vi "LIF V3.0.vi"() -> ()   [LabVIEW 2022 SP3]
uses:
  <vilib>/Utility/error.llb/DialogType.ctl
  <vilib>/DAQmx/read.llb/DAQmx Read (Analog 1D DBL 1Chan NSamp).vi
  <vilib>/DAQmx/create/channels.llb/DAQmx Create Channel (AI-Voltage-Basic).vi
  <vilib>/DAQmx/miscellaneous.llb/DAQmx Fill In Error Info.vi
  Instance           6 23Saved   Maxium LIF V2.0 .vi
  Instance           7 23Saved   Maxium LIF V2.0 .vi
  Instance           3 23Saved   Maxium LIF V2.0 .vi
panel:
  in  "Number of Samples to Average":i32=500
  out "Time Remaining":dbl format="%<%H:%M:%S>t"
  out "Scanning?":bool
  out "file ref":refnum<file>
  out "Sample X data":dbl[](array[numeric])
  out "sample Y data":dbl[](array[numeric])
  in  "STOP":bool
  out "Current Position (cm-1)":dbl format="%.3f"
  in  "Experimental Conditions":string
  in  "Time to wait (s)":dbl=6.0 min=0.0 max=60.0
  in  "Step Size (cm-1)":dbl=0.003 min=0.001 max=10.0 step=0.001 format="%.3f"
  in  "End Position (cm-1)":dbl=650.3 min=0.0 max=2000.0 step=0.001 format="%.3f"
  in  "Start Position (cm-1)":dbl min=0.0 max=0.0 step=0.001 format="%.3f"
  out "LIF Spectrum":cluster{"Y":dbl[], "Y":dbl[]}[](graph)
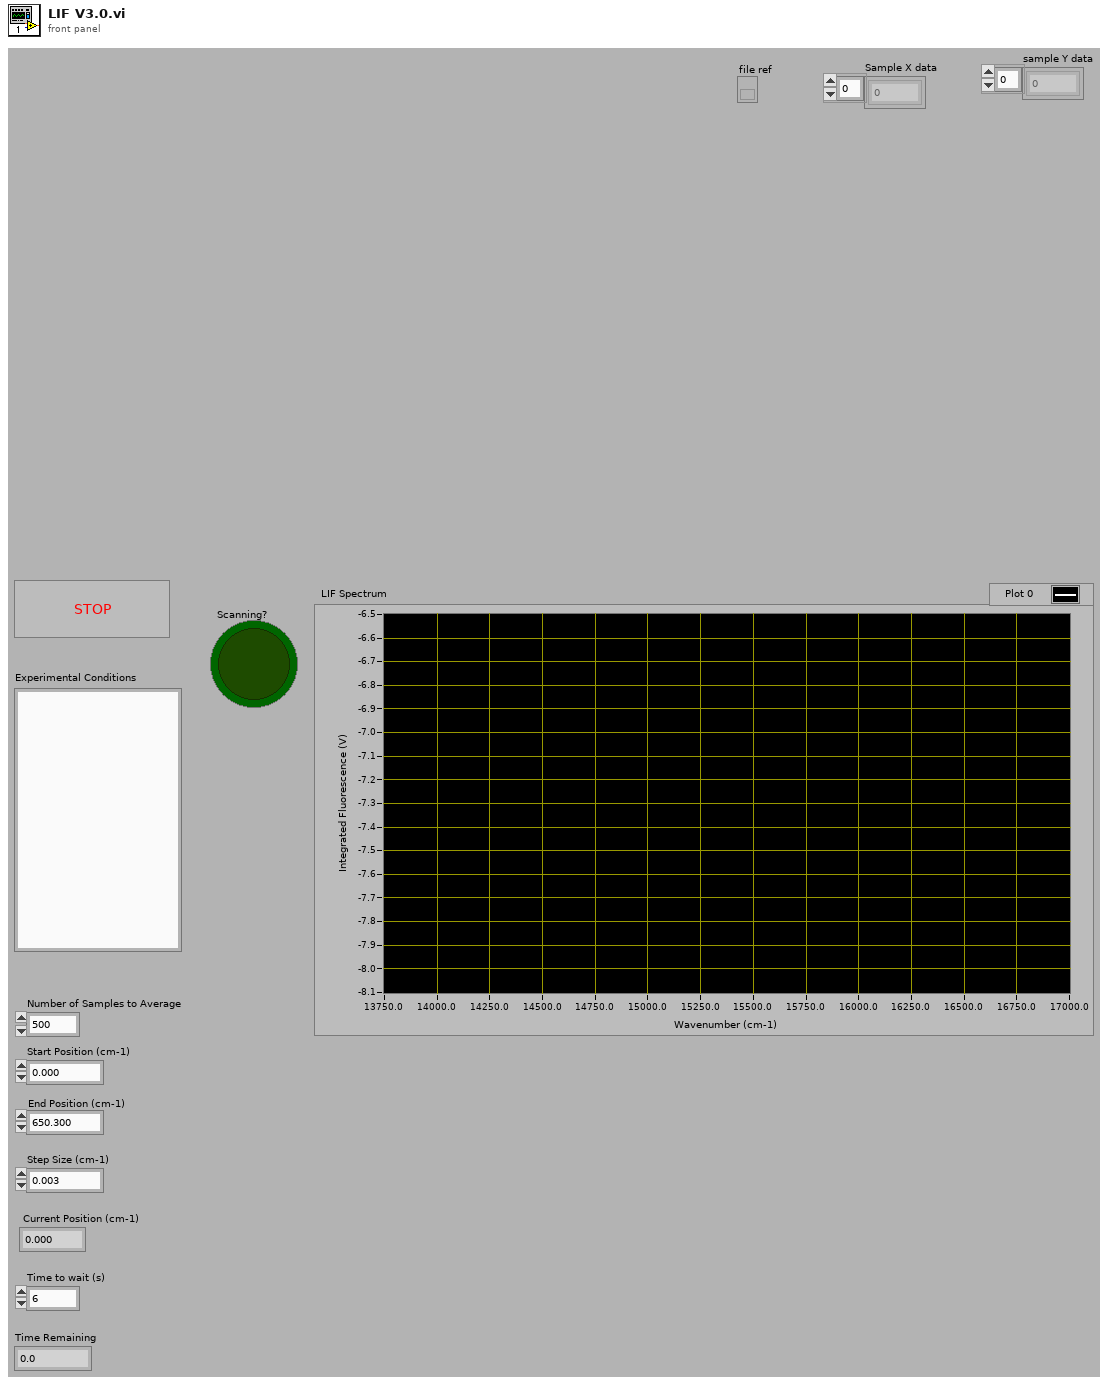
[diagram p1: front panel]
types:
  T1 = typedef "DialogType.ctl" = u16
  T2 = enum16{"open", "open or create", "create or replace", "create", "open (read only)"}
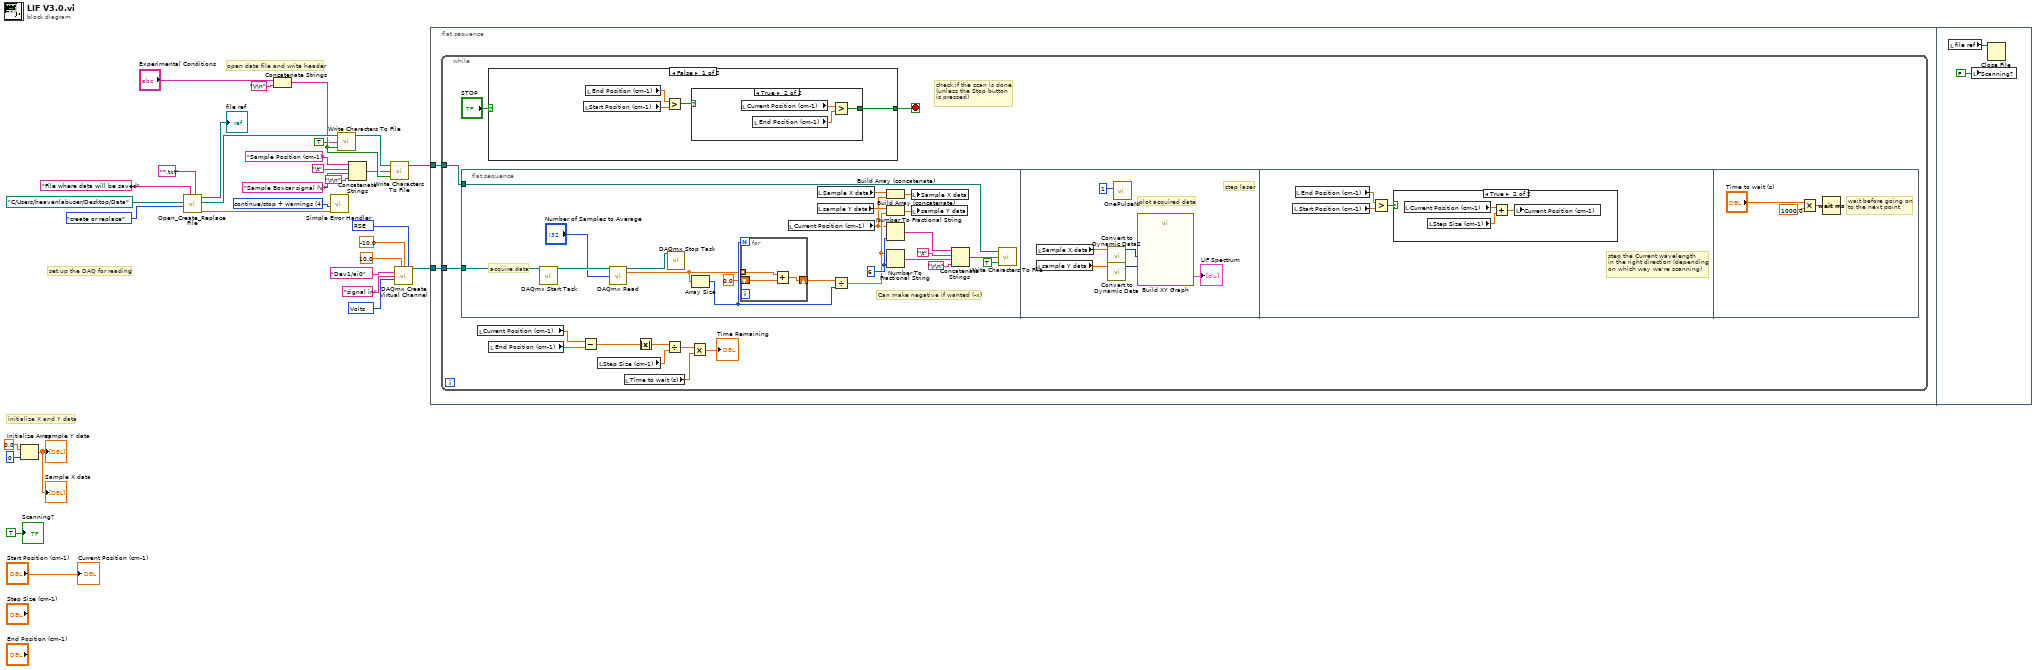
[diagram p0: block diagram]
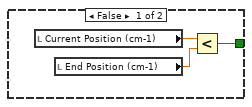
[diagram p2: hidden frame]
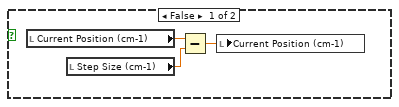
[diagram p4: hidden frame]
diagram:
  w14 = TRUE ("append to file? (new file:F)")
  w16 = T1 4 items=["no dialog", "OK message", "continue or stop message", "OK message + warnings", "continue/stop + warnings"] ("type of dialog (OK msg:1)")
  w26 = 10348 items=["Volts"=10348, "From Custom Scale"=10065] ("units")
  w31 = 10083 items=["default"=-1, "RSE"=10083, "NRSE"=10078, "Differential"=10106, "Pseudodifferential"=12529] ("input terminal configuration")
  # "open data file and write header"
  # "initialize X and Y data"
  # "set up the DAQ for reading"
  n1 = Initialize Array(0.0 ("element"), 0 ("dimension size")) -> (→"sample Y data" →"Sample X data":dbl[])
  n2 = call <vilib>:"Open_Create_Replace File.vi"("pattern"="*.txt", "prompt"="File where data will be saved", "function (open:0)"=T2."create or replace", "start path  (Not A Path)"=path "C:/Users/heavenlabuser/Desktop/Data") -> ("error out"=w17:errorcluster, "new file path"=w15:path, "refnum"=→"file ref":refnum<file>)  [unwired: 3 in, 2 out]
  n3 = Concatenate Strings("Experimental Conditions", "\r\n") -> (w10:string)
  n4 = call <vilib>:"Simple Error Handler.vi"("type of dialog (OK msg:1)"=w16, "error in (no error)"=w17) -> ()  [unwired: 1 in, 7 out]
  n5 = call <vilib>:"Write Characters To File.vi"("append to file? (new file:F)"=w14, "character string"=w10, "file path (dialog if empty)"=w15) -> ("new file path (Not A Path if cancelled)"=w13:path)  [unwired: 2 out]
  n6 = Concatenate Strings("Sample Position (cm-1)" ("string"), "\t", "Sample Boxcar signal (V)" ("string"), "\r\n") -> (w8:string)
  n7 = call <vilib>:"Write Characters To File.vi"("append to file? (new file:F)"=w14, "character string"=w8, "file path (dialog if empty)"=w13) -> ("new file path (Not A Path if cancelled)"=w7:path)  [unwired: 2 out]
  n8 = call-poly <vilib>:"DAQmx Create Virtual Channel.vi"("maximum value"=10.0, "minimum value"=-10.0, "input terminal configuration"=w31, "physical channels"=tag "Dev1/ai0", "name to assign"="signal in", "units"=w26) -> ("task out"=w2:refnum<k21>)  [unwired: 3 in, 6 out]
  n9 = flat-sequence {
    tunnel: w2 -> [w33]
    tunnel: w7 -> [w32]
    frame #0 {
      n10 = while {
        tunnel: w33 -> [w45]
        tunnel: w32 -> [w34]
        stop <- w43 stop-if-true
        # "check if the scan is done\n(unless the Stop button \nis pressed)"
        n11 = flat-sequence {
          tunnel: w45 -> [w74]
          tunnel: w34 -> [w68]
          frame #0 {
            w65 = i16 6 ("width (-)")
            # "Can make negative if wanted (-x)"
            # "acquire data"
            n12 = call <vilib>:"DAQmx Start Task.vi"("task/channels in"=w74) -> ("task out"=w73:refnum<k21>)  [unwired: 1 in, 13 out]
            n13 = call-poly <vilib>:"DAQmx Read.vi"("task/channels in"=w73, "number of samples per channel"="Number of Samples to Average") -> ("task out"=w72:refnum<k21>, "data"=w60:dbl[])  [unwired: 1 in, 11 out]
            n14 = call <vilib>:"DAQmx Stop Task.vi"("task/channels in"=w72) -> ()  [unwired: 1 in, 14 out]
            n15 = Array Size(array=w60) -> (size(s)=w64:i32)
            n16 = for {
              N: w64 -> [_]
              shift-right: [w80] -> w62
              shift-left: 0.0 ("y") -> [w81]
              tunnel: w60 -> [w79] mode=indexing
              n17 = Add(x=w79, y=w81) -> (x+y=w80:dbl)
            }
            n18 = local read "Current Position (cm-1)"() -> (w59:dbl)
            n19 = local read "Sample X data"() -> (w75:dbl[])
            n20 = local read "sample Y data"() -> (w77:dbl[])
            n21 = Divide(x=w62, y=w64) -> (x/y=w63:dbl)
            n22 = Build Array (concatenate)(w75, w59) -> (w76:dbl[])
            n23 = Build Array (concatenate)(w77, w63) -> (w78:dbl[])
            n24 = Number To Fractional String(number=w59, precision (6)=w65) -> (F-format string=w71:string)  [unwired: 2 out]
            n25 = Number To Fractional String(number=w63, precision (6)=w65) -> (F-format string=w69:string)  [unwired: 2 out]
            n26 = local write "Sample X data"(w76) -> ()
            n27 = local write "sample Y data"(w78) -> ()
            n28 = Concatenate Strings(w71, "\t", w69, "\r\n") -> (w67:string)
            n29 = call <vilib>:"Write Characters To File.vi"("append to file? (new file:F)"=TRUE, "character string"=w67, "file path (dialog if empty)"=w68) -> ()  [unwired: 3 out]
          }
          frame #1 {
            # "plot acquired data"
            # "step laser"
            n30 = local read "Sample X data"() -> (w84:dbl[])
            n31 = local read "sample Y data"() -> (w86:dbl[])
            n32 = call "Convert to Dynamic Data2"("Array"=w84) -> ("Dynamic Data Type"=w83:dynamicdata)  [unwired: 3 out]
            n33 = call "Convert to Dynamic Data"("Array"=w86) -> ("Dynamic Data Type"=w85:dynamicdata)  [unwired: 3 out]
            n34 = call "OnePulseNI.vi"("pulse width ms"=u32 1) -> ()  [unwired: 11 in]
            n35 = call "Build XY Graph"("Y Input"=w85, "X Input"=w83) -> ("XY Graph"=→"LIF Spectrum":cluster{"Y":dbl[], "Y":dbl[]}[])  [unwired: 3 in, 6 out]
          }
          frame #2 {
            # "step the Current wavelength\nin the right direction (depending\non which way we're scanning)"
            n36 = local read "Start Position (cm-1)"() -> (w89:dbl)
            n37 = local read "End Position (cm-1)"() -> (w88:dbl)
            n38 = Greater?(x=w88, y=w89) -> (0:w90:bool)
            n39 = case shown="True" w90 {
              frame False {
                n40 = local read "Current Position (cm-1)"() -> (w93:dbl)
                n41 = local read "Step Size (cm-1)"() -> (w92:dbl)
                n42 = Subtract(x=w93, y=w92) -> (x-y=w91:dbl)
                n43 = local write "Current Position (cm-1)"(w91) -> ()
              }
              frame True {
                n44 = local read "Current Position (cm-1)"() -> (w95:dbl)
                n45 = local read "Step Size (cm-1)"() -> (w94:dbl)
                n46 = Add(x=w95, y=w94) -> (x+y=w96:dbl)
                n47 = local write "Current Position (cm-1)"(w96) -> ()
              }
            }
          }
          frame #3 {
            # "wait before going on\nto the next point"
            n48 = Multiply(x="Time to wait (s)", y=1000.0) -> (x*y=w97:dbl)
            n49 = Wait (ms)(milliseconds to wait=w97) -> ()  [unwired: 1 out]
          }
        }
        n50 = local read "Current Position (cm-1)"() -> (w42:dbl)
        n51 = case shown="False" "STOP" {
          selector: "STOP" -> [_ w56]
          tunnel: [w49 w56] -> w43
          frame False {
            n52 = local read "Start Position (cm-1)"() -> (w47:dbl)
            n53 = local read "End Position (cm-1)"() -> (w48:dbl)
            n54 = Greater?(x=w48, y=w47) -> (0:w46:bool)
            n55 = case shown="True" w46 {
              tunnel: [w50 w55] -> w49
              frame False {
                n56 = local read "Current Position (cm-1)"() -> (w52:dbl)
                n57 = local read "End Position (cm-1)"() -> (w51:dbl)
                n58 = Less?(x=w52, y=w51) -> (x < y?=w50:bool)
              }
              frame True {
                n59 = local read "Current Position (cm-1)"() -> (w54:dbl)
                n60 = local read "End Position (cm-1)"() -> (w53:dbl)
                n61 = Greater?(x=w54, y=w53) -> (0:w55:bool)
              }
            }
          }
          frame True {
          }
        }
        n62 = local read "End Position (cm-1)"() -> (w41:dbl)
        n63 = Subtract(x=w42, y=w41) -> (x-y=w40:dbl)
        n64 = local read "Step Size (cm-1)"() -> (w38:dbl)
        n65 = local read "Time to wait (s)"() -> (w36:dbl)
        n66 = Absolute Value(x=w40) -> (abs(x)=w39:dbl)
        n67 = Divide(x=w39, y=w38) -> (x/y=w37:dbl)
        n68 = Multiply(x=w37, y=w36) -> (x*y=→"Time Remaining":dbl)
      }
    }
    frame #1 {
      n69 = local read "file ref"() -> (w101:refnum<file>)
      n70 = local write "Scanning?"(FALSE ("Scanning?")) -> ()
      n71 = Close File(refnum=w101) -> ()  [unwired: 1 in, 2 out]
    }
  }
  "Current Position (cm-1)" <- "Start Position (cm-1)"
  "Scanning?" <- TRUE ("Scanning?")
